vi "Ramp Pattern by Samples.vi"(6 "type":u16(ring) items=["Linear", "Logarithmic"], 8 "exclude end?":bool, 9 "start":dbl format="%0.2f", 10 "end":dbl=1.0 format="%0.2f", 11 "samples":i32=128) -> (0 "error":i32, 3 "Ramp Pattern":dbl[](array[numeric]))   [LabVIEW 2020, in "NI_AALBase.lvlib"]
doc: "Generates an array containing a ramp pattern. You must manually select the polymorphic instance you want to use."
uses:
  NI_AALBase.lvlib
  <resource>/lvanlys.dll
panel:
  # "Ramp Pattern"
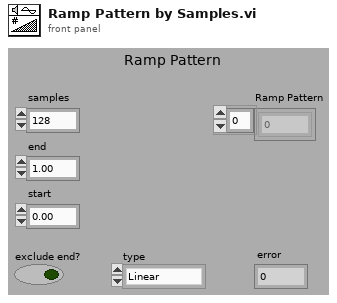
[diagram p1: front panel]
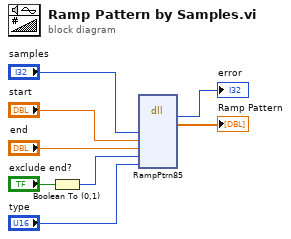
[diagram p0: block diagram]
diagram:
  n1 = Boolean To (0,1)(Boolean="exclude end?") -> (0, 1=w3:i16)
  n2 = dll-call lib="C:/Program Files/National Instruments/LabVIEW 2020/resource/lvanlys.*" fn="RampPtrn85"("size"="samples", "start"="start", "end"="end", "noEnd"=w3, "type"="type") -> ("return type"=→"error":i32, "Ramp Pattern"=→"Ramp Pattern":dbl[])  [unwired: 9 in, 2 out]
